vi "Set TCP Ports.vi"(8 "error in (no error)":errorcluster, 11 "Cfg Grandmaster in":refnum<class "Cfg Grandmaster.lvclass">) -> (0 "error out":errorcluster, 3 "Cfg Grandmaster out":refnum<class "Cfg Grandmaster.lvclass">)   [LabVIEW 2018, in "Configuration Grandmaster.lvlib" / "Cfg Grandmaster.lvclass"]
uses:
  Cfg Grandmaster.lvclass
  Cfg Grandmaster.lvclass/Cfg Grandmaster.ctl
  TCP Server/TCP Connection Messages/Update Port Msg/Update Port Msg.lvclass/Update Port Msg.ctl
  <vilib>/ActorFramework/Message Enqueuer/Message Enqueuer.lvclass/Message Enqueuer.ctl
  <vilib>/ActorFramework/Message Enqueuer/Enqueue.vi
  TCP Server/TCP Connection Messages/Update Port Msg/Update Port Msg.lvclass
  C:/Program Files (x86)/National Instruments/LabVIEW 2018/vi.lib/ActorFramework/Message/Message.lvclass
  <vilib>/ActorFramework/Message Priority Queue/Priority Enqueue.vi
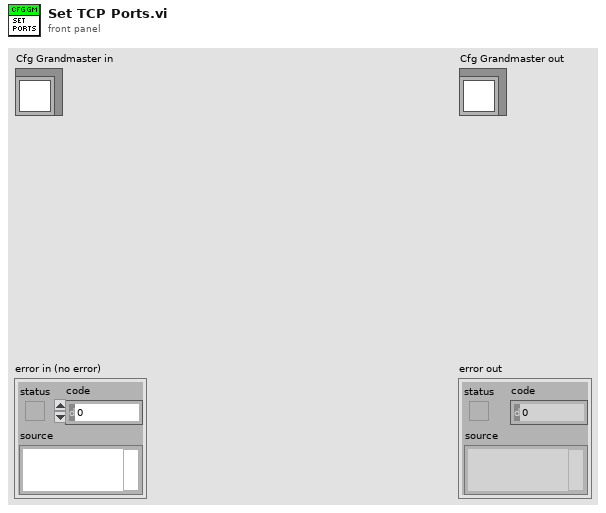
[diagram p1: front panel]
types:
  T1 = typedef "TCP Ports.ctl" = cluster{"Port Rdr":u16, "Port HS":u16, "Port LS":u16}
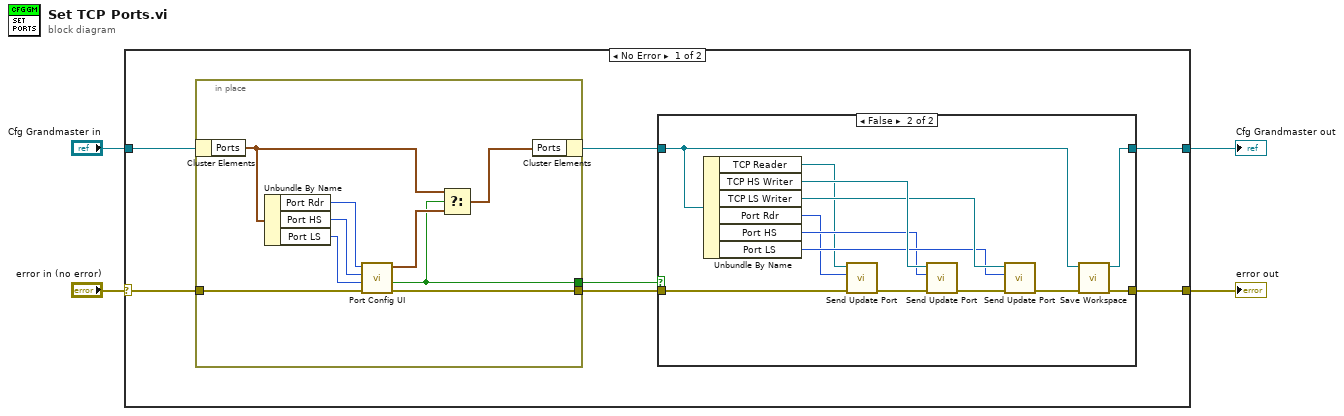
[diagram p0: block diagram]
diagram:
  n1 = case shown="No Error" "error in (no error)" {
    selector: "error in (no error)" -> [w11 w37]
    tunnel: [w8 w37] -> w3
    tunnel: [w6 w36] -> w1
    tunnel: "Cfg Grandmaster in" -> [w10 w36]
    frame No Error {
      n2 = in-place {
        in-place-border: [w30] -> w9
        in-place-border: w11 -> [w35]
        in-place-border: [w31] -> w5
        n3 = in-place-cluster #1(w10) -> ("Ports"=w34:T1)
        n4 = Unbundle By Name(w34) -> ("Port Rdr"=w27:u16, "Port HS"=w28:u16, "Port LS"=w29:u16)
        n5 = call "Port Config UI.vi"("error in (no error)"=w35, "Port LS"=w29, "Port HS"=w28, "Port Rdr"=w27) -> ("error out"=w30:errorcluster, "Canceled?"=w31:bool, "Ports"=w33:T1)  [unwired: 5 in]
        n6 = Select(t=w34, s=w31, f=w33) -> (s? t:f=w32:T1)
        n7 = in-place-cluster #1("Ports"=w32) -> (w7:refnum<class "Cfg Grandmaster.lvclass">)
      }
      n8 = case shown="False" w5 {
        tunnel: w9 -> [w12 w16]
        tunnel: [w12 w26] -> w8
        tunnel: w7 -> [w13 w22]
        tunnel: [w13 w25] -> w6
        frame True {
        }
        frame False {
          n9 = Unbundle By Name(w22) -> ("TCP Reader"=w15:refnum<class "Message Enqueuer.lvclass">, "TCP HS Writer"=w21:refnum<class "Message Enqueuer.lvclass">, "TCP LS Writer"=w20:refnum<class "Message Enqueuer.lvclass">, "Port Rdr"=w14:u16, "Port HS"=w18:u16, "Port LS"=w19:u16)
          n10 = call "Send Update Port.vi"("error in (no error)"=w16, "Port"=w14, "Message Enqueuer"=w15) -> ("error out"=w17:errorcluster)  [unwired: 7 in, 1 out]
          n11 = call "Send Update Port.vi"("error in (no error)"=w17, "Port"=w18, "Message Enqueuer"=w21) -> ("error out"=w23:errorcluster)  [unwired: 7 in, 1 out]
          n12 = call "Send Update Port.vi"("error in (no error)"=w23, "Port"=w19, "Message Enqueuer"=w20) -> ("error out"=w24:errorcluster)  [unwired: 7 in, 1 out]
          n13 = call "Save Workspace.vi"("error in (no error)"=w24, "Cfg Grandmaster in"=w22) -> ("error out"=w26:errorcluster, "Cfg Grandmaster out"=w25:refnum<class "Cfg Grandmaster.lvclass">)  [unwired: 8 in]
        }
      }
    }
    frame Error {
    }
  }
  "error out" <- w3
  "Cfg Grandmaster out" <- w1
